vi "USB6343_Control_v1.6.vi"(8 "error in":errorcluster caption="错误输出") -> (0 "error out":errorcluster caption="错误输出")   [LabVIEW 2013]
uses:
  <vilib>/DAQmx/read.llb/DAQmx Read (Analog 1D DBL NChan 1Samp).vi
  <vilib>/DAQmx/read.llb/DAQmx Read (Digital 1D Bool NChan 1Samp 1Line).vi
  <vilib>/DAQmx/read.llb/DAQmx Read (Counter DBL 1Chan 1Samp).vi
  <vilib>/DAQmx/write.llb/DAQmx Write (Digital 1D Bool NChan 1Samp 1Line).vi
  <vilib>/DAQmx/write.llb/DAQmx Write (Analog 1D DBL NChan 1Samp).vi
  <vilib>/DAQmx/miscellaneous.llb/DAQmx Fill In Error Info.vi
  current_position.vi
  <vilib>/DAQmx/configure/timing.llb/DAQmx Timing (Implicit).vi
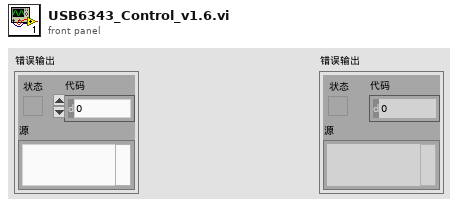
[diagram p1: front panel]
types:
  T1 = typedef "Semaphore RefNum" = refnum<k1>
  T2 = cluster{"monitor":refnum<user-event>, "motor status":refnum<user-event>, "motor":refnum<user-event>, "notifier out":refnum<notifier>, "queue out":refnum<queue>, "AI":T1, "DI":T1, "CX":T1, "CY":T1}
  T3 = cluster{"AI Task":refnum<k21>, "AO Task":refnum<k21>, "DO Task":refnum<k21>, "DI Task":refnum<k21>, "PWM x":refnum<k21>, "PWM y":refnum<k21>, "counter x":refnum<k21>, "counter y":refnum<k21>}
  T4 = cluster{"cmd":string, "channel":i32, "value":dbl, "on/off":bool, "return value":refnum<vi>}
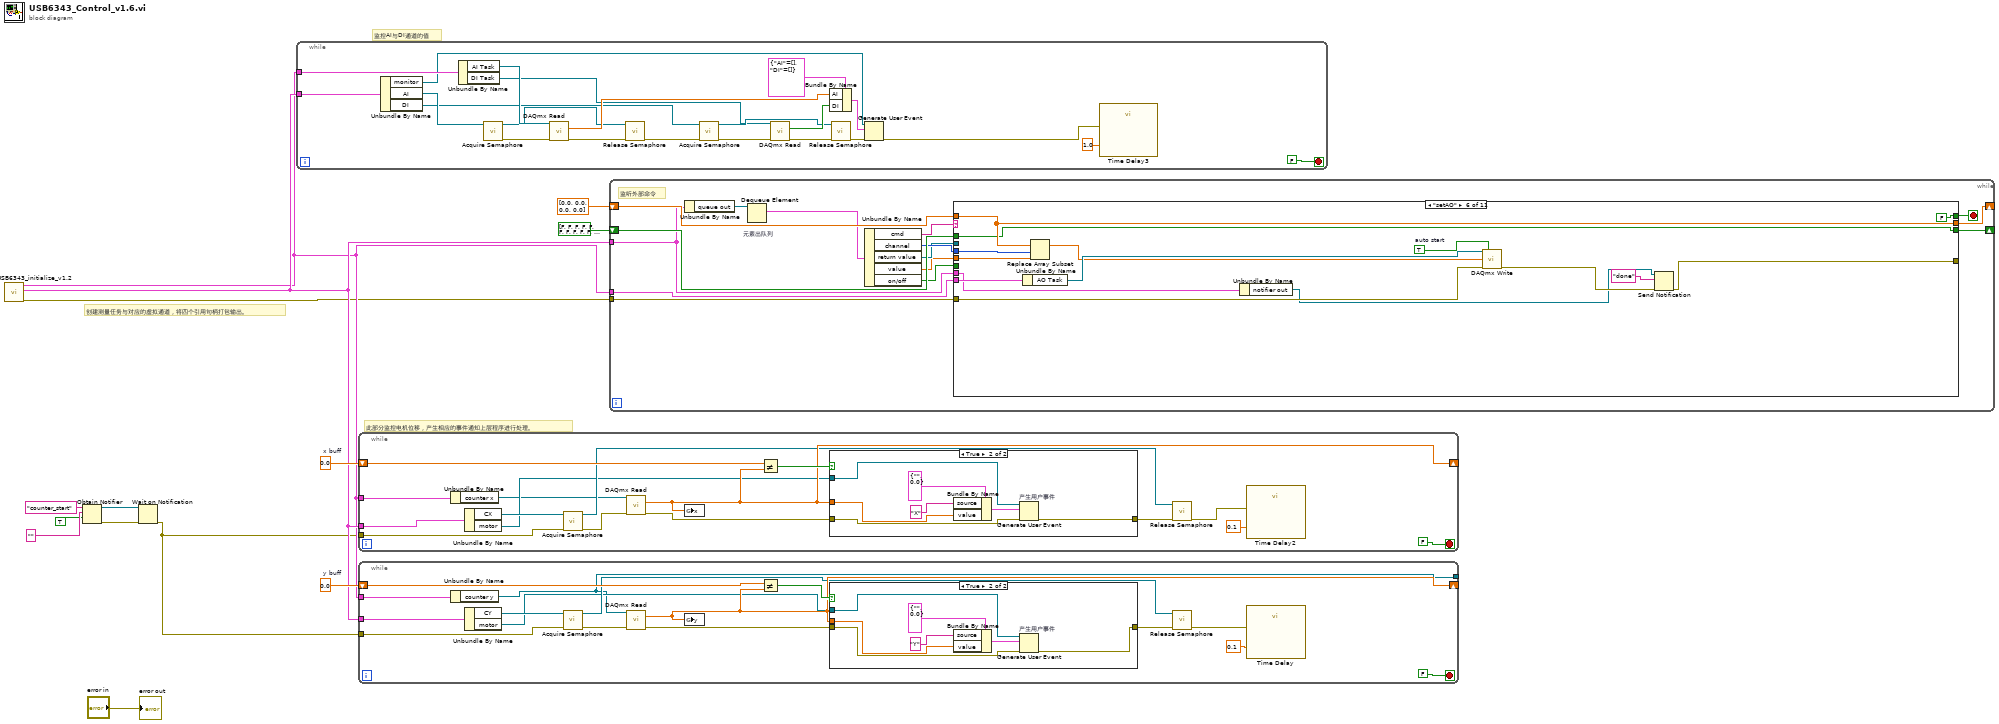
[diagram p0: block diagram]
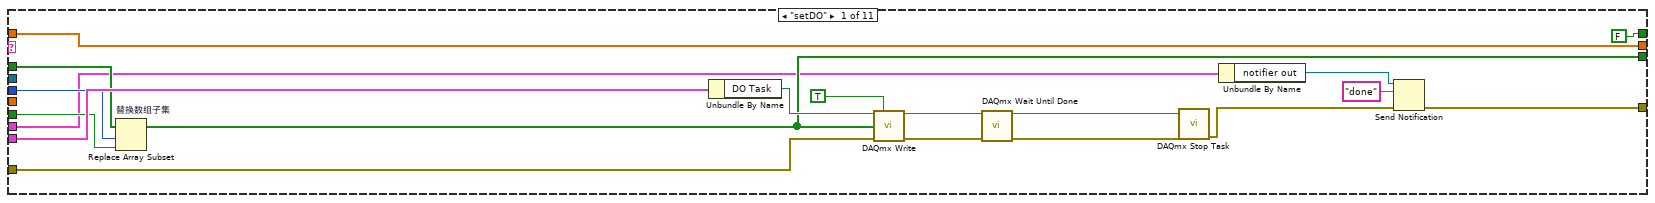
[diagram p4: hidden frame]
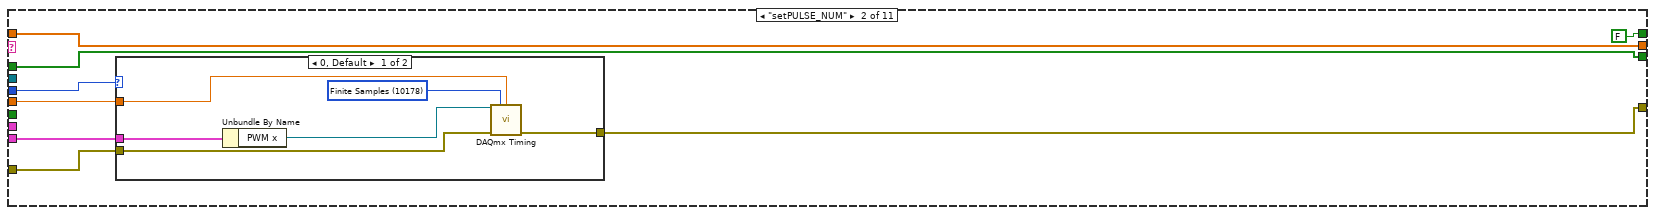
[diagram p5: hidden frame]
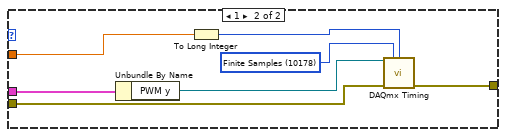
[diagram p6: hidden frame]
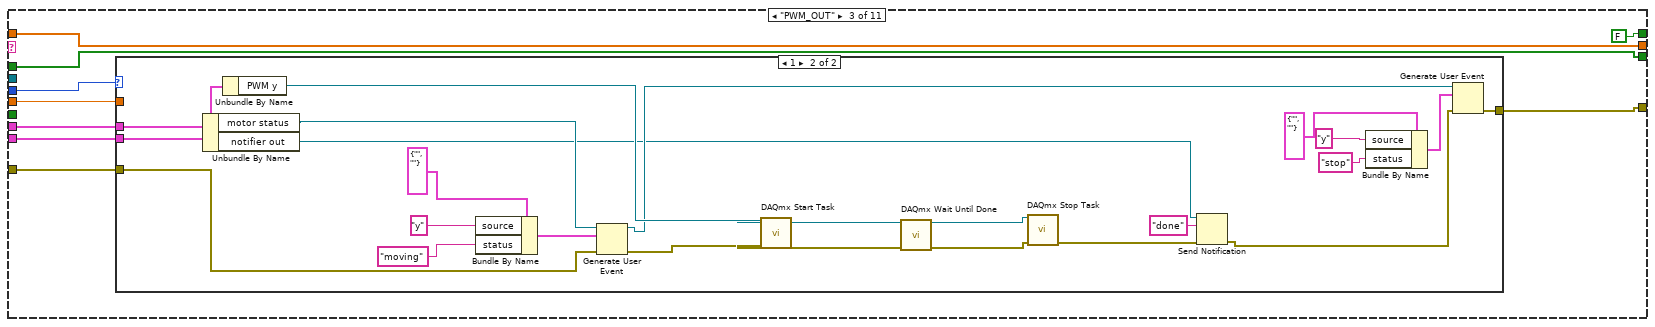
[diagram p7: hidden frame]
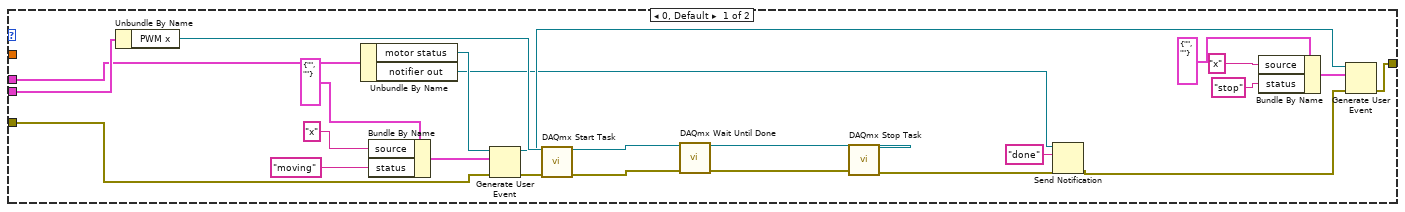
[diagram p8: hidden frame]
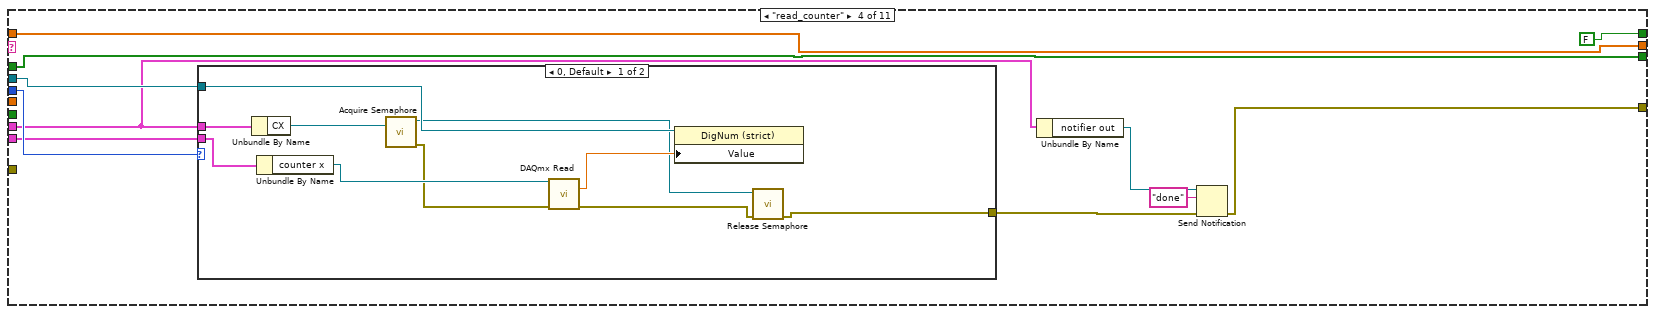
[diagram p9: hidden frame]
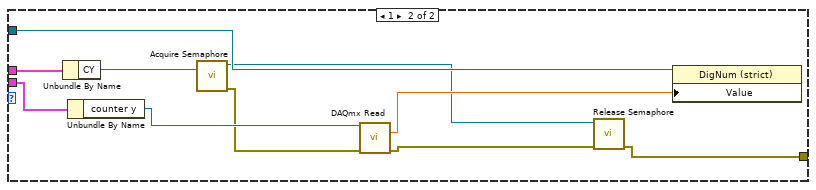
[diagram p10: hidden frame]
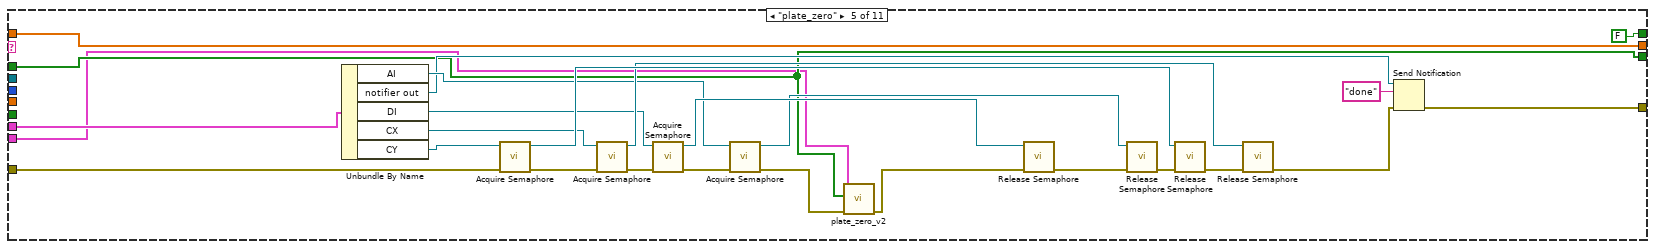
[diagram p11: hidden frame]
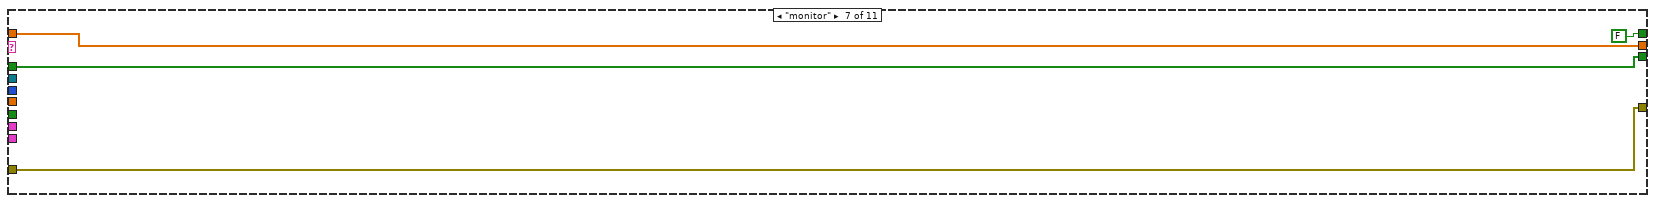
[diagram p12: hidden frame]
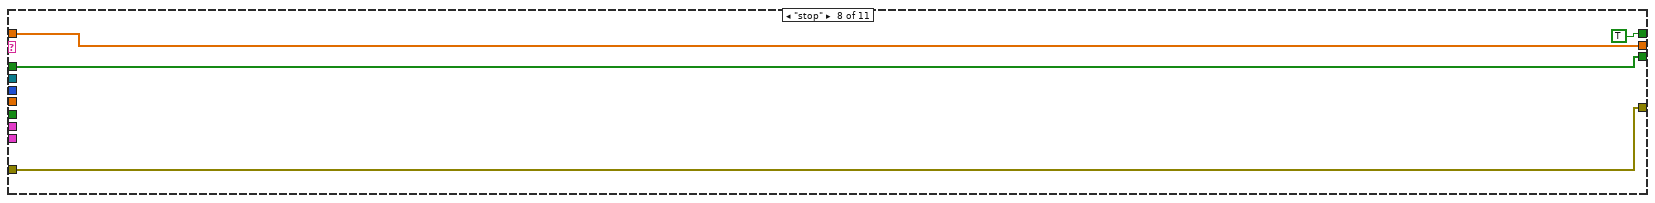
[diagram p13: hidden frame]
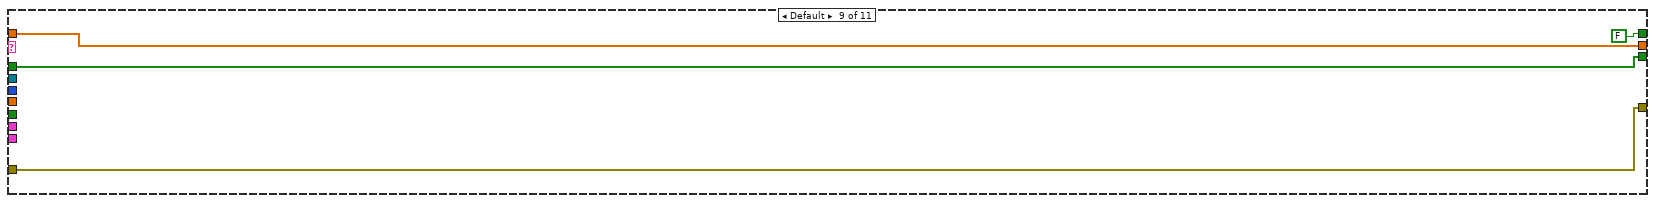
[diagram p14: hidden frame]
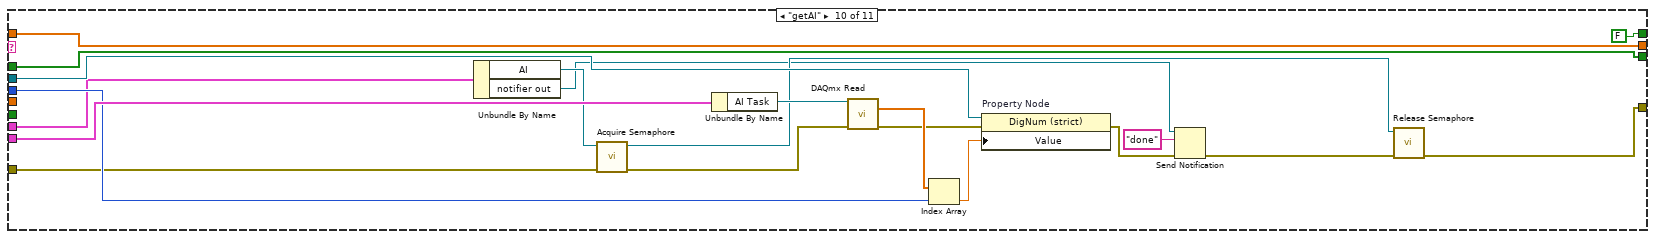
[diagram p15: hidden frame]
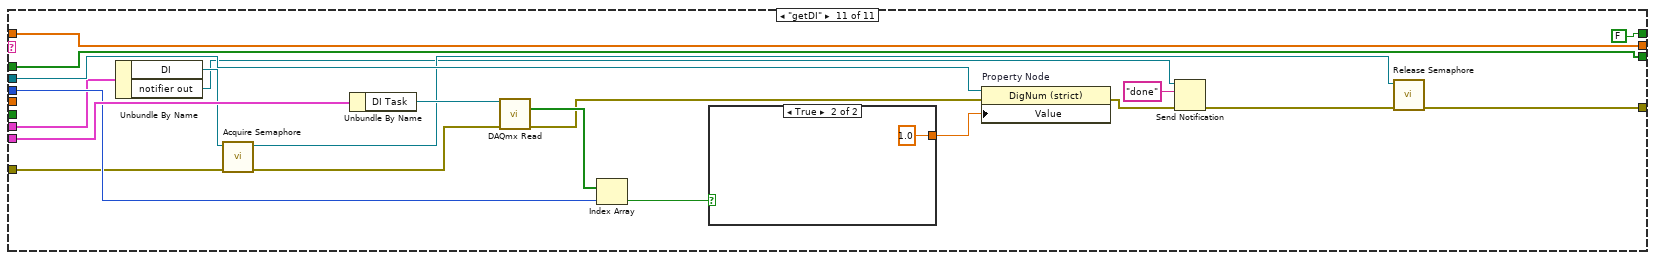
[diagram p16: hidden frame]
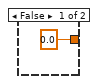
[diagram p17: hidden frame]
diagram:
  w11 = 0.0  # x buff
  w12 = 0.0  # y buff
  # "监控AI与DI通道的值"
  # "此部分监控电机位移，产生相应的事件通知上层程序进行处理。"
  # "创建测量任务与对应的虚拟通道，将四个引用句柄打包输出。"
  n1 = call "USB6343_initialize_v1.2.vi"() -> ("error out"=w7:errorcluster, "interface"=w10:T2, "tasks"=w9:T3)  [unwired: 9 in]
  n2 = Obtain Notifier(name (unnamed)="counter_start", notification data type="", create if not found? (T)=TRUE) -> (notifier out=w3:refnum<notifier>, error out=w4:errorcluster)  [unwired: 1 in, 1 out]
  n3 = Wait on Notification(notifier=w3, error in (no error)=w4) -> (error out=w2:errorcluster)  [unwired: 2 in, 3 out]
  n4 = while {
    tunnel: w9 -> [w34]
    tunnel: w10 -> [w19]
    stop <- FALSE stop-if-true
    n5 = Unbundle By Name(w19) -> ("monitor"=w18:refnum<user-event>, "AI"=w17:T1, "DI"=w16:T1)
    n6 = Unbundle By Name(w34) -> ("AI Task"=w35:refnum<k21>, "DI Task"=w15:refnum<k21>)
    n7 = call <vilib>:"Acquire Semaphore.vi"("semaphore"=w17) -> ("error out"=w20:errorcluster, "semaphore out"=w22:T1)  [unwired: 4 in, 1 out]
    n8 = call-poly <vilib>:"DAQmx Read.vi"("task/channels in"=w35, "error in"=w20) -> ("data"=w32:dbl[], "error out"=w27:errorcluster)  [unwired: 11 in, 1 out]
    n9 = call <vilib>:"Release Semaphore.vi"("error in (no error)"=w27, "semaphore"=w22) -> ("error out"=w26:errorcluster)  [unwired: 4 in, 1 out]
    n10 = call <vilib>:"Acquire Semaphore.vi"("error in (no error)"=w26, "semaphore"=w16) -> ("error out"=w25:errorcluster, "semaphore out"=w21:T1)  [unwired: 3 in, 1 out]
    n11 = call-poly <vilib>:"DAQmx Read.vi"("task/channels in"=w15, "error in"=w25) -> ("data"=w31:bool[], "error out"=w24:errorcluster)  [unwired: 11 in, 1 out]
    n12 = Bundle By Name(cluster=cluster{"AI":dbl[], "DI":bool[]} {"AI"=[], "DI"=[]} ("event data"), "AI"=w32, "DI"=w31) -> (w28:cluster{"AI":dbl[], "DI":bool[]})
    n13 = call <vilib>:"Release Semaphore.vi"("error in (no error)"=w24, "semaphore"=w21) -> ("error out"=w23:errorcluster)  [unwired: 4 in, 1 out]
    n14 = Generate User Event(user event=w18, event data cluster=w28, error in=w23) -> (error out=w30:errorcluster)  [unwired: 1 in, 1 out]
    n15 = call "Time Delay3"("error in (no error)"=w30, "Delay Time (s)"=1.0) -> ()  [unwired: 9 in, 1 out]
  }
  n16 = while {
    shift-right: [w48] -> _
    shift-left: w11 -> [w52]
    tunnel: w10 -> [w42]
    tunnel: w9 -> [w39]
    tunnel: w2 -> [w37]
    stop <- FALSE stop-if-true
    n17 = Unbundle By Name(w39) -> ("counter x"=w38:refnum<k21>)
    n18 = Unbundle By Name(w42) -> ("CX"=w41:T1, "motor"=w40:refnum<user-event>)
    n19 = call <vilib>:"Acquire Semaphore.vi"("error in (no error)"=w37, "semaphore"=w41) -> ("error out"=w47:errorcluster, "semaphore out"=w44:T1)  [unwired: 3 in, 1 out]
    n20 = call-poly <vilib>:"DAQmx Read.vi"("task/channels in"=w38, "error in"=w47) -> ("data"=w48:dbl, "error out"=w50:errorcluster)  [unwired: 11 in, 1 out]
    n21 = global write "current_position.vi" "x"(w48) -> ()
    n22 = Not Equal?(x=w52, y=w48) -> (x != y?=w51:bool)
    n23 = case shown="True" w51 {
      tunnel: w48 -> [_ w54]
      tunnel: w50 -> [w53 w57]
      tunnel: [w53 w56] -> w46
      tunnel: w40 -> [_ w55]
      frame False {
      }
      frame True {
        n24 = Bundle By Name(cluster=cluster{"source":string, "value":dbl} {"source"="", "value"=0.0} ("事件数据"), "source"="X", "value"=w54) -> (w58:cluster{"source":string, "value":dbl})
        n25 = Generate User Event "产生用户事件"(user event=w55, event data cluster=w58, error in=w57) -> (error out=w56:errorcluster)  [unwired: 1 in, 1 out]
      }
    }
    n26 = call <vilib>:"Release Semaphore.vi"("error in (no error)"=w46, "semaphore"=w44) -> ("error out"=w45:errorcluster)  [unwired: 4 in, 1 out]
    n27 = call "Time Delay2"("error in (no error)"=w45, "Delay Time (s)"=0.1) -> ()  [unwired: 9 in, 1 out]
  }
  n28 = while {
    tunnel: [w62] -> _
    shift-right: [w72] -> _
    shift-left: w12 -> [w76]
    tunnel: w10 -> [w66]
    tunnel: w9 -> [w63]
    tunnel: w2 -> [w61]
    stop <- FALSE stop-if-true
    n29 = Unbundle By Name(w63) -> ("counter y"=w62:refnum<k21>)
    n30 = Unbundle By Name(w66) -> ("CY"=w65:T1, "motor"=w64:refnum<user-event>)
    n31 = call <vilib>:"Acquire Semaphore.vi"("error in (no error)"=w61, "semaphore"=w65) -> ("error out"=w71:errorcluster, "semaphore out"=w68:T1)  [unwired: 3 in, 1 out]
    n32 = call-poly <vilib>:"DAQmx Read.vi"("task/channels in"=w62, "error in"=w71) -> ("data"=w72:dbl, "error out"=w74:errorcluster)  [unwired: 11 in, 1 out]
    n33 = global write "current_position.vi" "y"(w72) -> ()
    n34 = Not Equal?(x=w76, y=w72) -> (x != y?=w75:bool)
    n35 = case shown="True" w75 {
      tunnel: w72 -> [_ w78]
      tunnel: w74 -> [w77 w80]
      tunnel: [w77 w79] -> w70
      tunnel: w64 -> [_ w81]
      frame False {
      }
      frame True {
        n36 = Bundle By Name(cluster=cluster{"source":string, "value":dbl} {"source"="", "value"=0.0} ("事件数据"), "source"="Y", "value"=w78) -> (w82:cluster{"source":string, "value":dbl})
        n37 = Generate User Event "产生用户事件"(user event=w81, event data cluster=w82, error in=w80) -> (error out=w79:errorcluster)  [unwired: 1 in, 1 out]
      }
    }
    n38 = call <vilib>:"Release Semaphore.vi"("error in (no error)"=w70, "semaphore"=w68) -> ("error out"=w69:errorcluster)  [unwired: 4 in, 1 out]
    n39 = call "Time Delay"("error in (no error)"=w69, "Delay Time (s)"=0.1) -> ()  [unwired: 9 in, 1 out]
  }
  n40 = while {
    tunnel: w9 -> [w93]
    tunnel: w7 -> [w99]
    shift-right: [w97] -> _
    shift-left: bool[] [FALSE, FALSE, FALSE, FALSE, FALSE, FALSE, FALSE, FALSE, FALSE, FALSE, FALSE, FALSE, FALSE, FALSE, FALSE, FALSE] -> [w98]
    shift-right: [w94] -> _
    shift-left: dbl[] [0.0, 0.0, 0.0, 0.0] ("data") -> [w95]
    tunnel: w10 -> [w86]
    stop <- w96 stop-if-true
    # "监听外部命令"
    n41 = Unbundle By Name(w86) -> ("queue out"=w85:refnum<queue>)
    n42 = Dequeue Element "元素出队列"(queue=w85) -> (element=w92:T4)  [unwired: 2 in, 3 out]
    n43 = Unbundle By Name(w92) -> ("cmd"=w91:string, "channel"=w90:i32, "return value"=w89:refnum<vi>, "value"=w87:dbl, "on/off"=w88:bool)
    n44 = case shown="\"setAO\"" w91 {
      tunnel: w90 -> [w116 w120 w142 w207 _ w266 _ _ _ w296 w319]
      tunnel: w93 -> [w118 w123 w145 w206 w229 w268 _ _ _ w300 w321]
      tunnel: w99 -> [w110 w121 w143 _ w245 w260 w269 w273 w277 w289 w309]
      tunnel: w98 -> [w117 w124 w146 w197 w231 w264 w272 w276 w280 w294 w318]
      tunnel: w88 -> [w115 _ _ _ _ _ _ _ _ _ _]
      tunnel: [w108 w124 w146 w197 w231 w264 w272 w276 w280 w294 w318] -> w97
      tunnel: [FALSE FALSE FALSE FALSE FALSE FALSE FALSE TRUE FALSE FALSE FALSE] -> w96
      tunnel: w95 -> [w113 w125 w147 w198 w252 w265 w271 w274 w278 w293 w317]
      tunnel: [w113 w125 w147 w198 w252 w265 w271 w274 w278 w293 w317] -> w94
      tunnel: w89 -> [_ _ _ w205 _ _ _ _ _ w298 w320]
      tunnel: [w112 w119 w141 w200 w251 w257 w269 w273 w277 w285 w304] -> _
      tunnel: w87 -> [_ w122 w144 _ _ w259 _ _ _ _ _]
      tunnel: w86 -> [w104 _ w140 w203 w237 w256 _ _ _ w283 w303]
      frame "setDO" {
        n45 = Replace Array Subset "替换数组子集"(array=w117, new element=w115, index=w116) -> (w108:bool[])
        n46 = Unbundle By Name(w118) -> ("DO Task"=w109:refnum<k21>)
        n47 = call-poly <vilib>:"DAQmx Write.vi"("task/channels in"=w109, "auto start"=TRUE, "data"=w108, "error in"=w110) -> ("task out"=w105:refnum<k21>, "error out"=w106:errorcluster)  [unwired: 9 in, 1 out]
        n48 = call <vilib>:"DAQmx Wait Until Done.vi"("task/channels in"=w105, "error in"=w106) -> ("task out"=w100:refnum<k21>, "error out"=w102:errorcluster)  [unwired: 12 in]
        n49 = call <vilib>:"DAQmx Stop Task.vi"("task/channels in"=w100, "error in"=w102) -> ("error out"=w101:errorcluster)  [unwired: 12 in, 1 out]
        n50 = Unbundle By Name(w104) -> ("notifier out"=w103:refnum<notifier>)
        n51 = Send Notification(notification="done" ("通知"), notifier=w103, error in (no error)=w101) -> (error out=w112:errorcluster)  [unwired: 1 out]
      }
      frame "setPULSE_NUM" {
        n52 = case shown="0, Default" w120 {
          tunnel: w123 -> [w132 w139]
          tunnel: w122 -> [w129 w134]
          tunnel: w121 -> [w128 w136]
          tunnel: [w127 w135] -> w119
          frame 0, Default {
            w130 = 10178 items=["Finite Samples"=10178, "Continuous Samples"=10123, "Hardware Timed Single Point"=12522] ("sample mode")
            n53 = Unbundle By Name(w132) -> ("PWM x"=w131:refnum<k21>)
            n54 = call-poly <vilib>:"DAQmx Timing.vi"("task/channels in"=w131, "sample mode"=w130, "samples per channel"=w129, "error in"=w128) -> ("error out"=w127:errorcluster)  [unwired: 10 in, 1 out]
          }
          frame 1 {
            w137 = 10178 items=["Finite Samples"=10178, "Continuous Samples"=10123, "Hardware Timed Single Point"=12522] ("sample mode")
            n55 = Unbundle By Name(w139) -> ("PWM y"=w138:refnum<k21>)
            n56 = To Long Integer(number=w134) -> (32bit integer=w133:i32)
            n57 = call-poly <vilib>:"DAQmx Timing.vi"("task/channels in"=w138, "sample mode"=w137, "samples per channel"=w133, "error in"=w136) -> ("error out"=w135:errorcluster)  [unwired: 10 in, 1 out]
          }
        }
      }
      frame "PWM_OUT" {
        n58 = case shown="1" w142 {
          tunnel: w145 -> [w172 w196]
          tunnel: w144 -> [_ _]
          tunnel: w143 -> [w164 w188]
          tunnel: [w157 w182] -> w141
          tunnel: w140 -> [w155 w179]
          frame 0, Default {
            n59 = Unbundle By Name(w172) -> ("PWM x"=w171:refnum<k21>)
            n60 = Unbundle By Name(w155) -> ("motor status"=w154:refnum<user-event>, "notifier out"=w149:refnum<notifier>)
            n61 = Bundle By Name(cluster=cluster{"source":string, " status":string} {"source"="", " status"=""} ("event data"), "source"="x", "status"="moving") -> (w162:cluster{"source":string, " status":string})
            n62 = Generate User Event(user event=w154, event data cluster=w162, error in=w164) -> (user event out=w156:refnum<user-event>, error out=w163:errorcluster)  [unwired: 1 in]
            n63 = call <vilib>:"DAQmx Start Task.vi"("task/channels in"=w171, "error in"=w163) -> ("task out"=w169:refnum<k21>, "error out"=w170:errorcluster)  [unwired: 12 in]
            n64 = call <vilib>:"DAQmx Wait Until Done.vi"("task/channels in"=w169, "error in"=w170) -> ("task out"=w168:refnum<k21>, "error out"=w153:errorcluster)  [unwired: 12 in]
            n65 = call <vilib>:"DAQmx Stop Task.vi"("task/channels in"=w168, "error in"=w153) -> ("error out"=w152:errorcluster)  [unwired: 12 in, 1 out]
            n66 = Send Notification(notification="done", notifier=w149, error in (no error)=w152) -> (error out=w151:errorcluster)  [unwired: 1 out]
            n67 = Bundle By Name(cluster=cluster{"source":string, " status":string} {"source"="", " status"=""} ("event data"), "source"="x", "status"="stop") -> (w158:cluster{"source":string, " status":string})
            n68 = Generate User Event(user event=w156, event data cluster=w158, error in=w151) -> (error out=w157:errorcluster)  [unwired: 1 in, 1 out]
          }
          frame 1 {
            n69 = Unbundle By Name(w179) -> ("motor status"=w178:refnum<user-event>, "notifier out"=w173:refnum<notifier>)
            n70 = Unbundle By Name(w196) -> ("PWM y"=w195:refnum<k21>)
            n71 = Bundle By Name(cluster=cluster{"source":string, " status":string} {"source"="", " status"=""} ("event data"), "source"="y", "status"="moving") -> (w181:cluster{"source":string, " status":string})
            n72 = Generate User Event(user event=w178, event data cluster=w181, error in=w188) -> (user event out=w177:refnum<user-event>, error out=w187:errorcluster)  [unwired: 1 in]
            n73 = call <vilib>:"DAQmx Start Task.vi"("task/channels in"=w195, "error in"=w187) -> ("task out"=w193:refnum<k21>, "error out"=w194:errorcluster)  [unwired: 12 in]
            n74 = call <vilib>:"DAQmx Wait Until Done.vi"("task/channels in"=w193, "error in"=w194) -> ("task out"=w191:refnum<k21>, "error out"=w192:errorcluster)  [unwired: 12 in]
            n75 = call <vilib>:"DAQmx Stop Task.vi"("task/channels in"=w191, "error in"=w192) -> ("error out"=w176:errorcluster)  [unwired: 12 in, 1 out]
            n76 = Send Notification(notification="done", notifier=w173, error in (no error)=w176) -> (error out=w175:errorcluster)  [unwired: 1 out]
            n77 = Bundle By Name(cluster=cluster{"source":string, " status":string} {"source"="", " status"=""} ("event data"), "source"="y", "status"="stop") -> (w183:cluster{"source":string, " status":string})
            n78 = Generate User Event(user event=w177, event data cluster=w183, error in=w175) -> (error out=w182:errorcluster)  [unwired: 1 in, 1 out]
          }
        }
      }
      frame "read_counter" {
        n79 = case shown="0, Default" w207 {
          tunnel: w203 -> [w217 w227]
          tunnel: w206 -> [w215 w225]
          tunnel: w205 -> [w212 w222]
          tunnel: [w208 w218] -> w204
          frame 0, Default {
            n80 = Unbundle By Name(w217) -> ("CX"=w216:T1)
            n81 = Unbundle By Name(w215) -> ("counter x"=w214:refnum<k21>)
            n82 = call <vilib>:"Acquire Semaphore.vi"("semaphore"=w216) -> ("error out"=w213:errorcluster, "semaphore out"=w209:T1)  [unwired: 4 in, 1 out]
            n83 = call-poly <vilib>:"DAQmx Read.vi"("task/channels in"=w214, "error in"=w213) -> ("data"=w211:dbl, "error out"=w210:errorcluster)  [unwired: 11 in, 1 out]
            n84 = property class="DigNum (strict)"(reference=w212, "Value"=w211) -> ()  [unwired: 1 in, 2 out]
            n85 = call <vilib>:"Release Semaphore.vi"("error in (no error)"=w210, "semaphore"=w209) -> ("error out"=w208:errorcluster)  [unwired: 4 in, 1 out]
          }
          frame 1 {
            n86 = Unbundle By Name(w227) -> ("CY"=w226:T1)
            n87 = Unbundle By Name(w225) -> ("counter y"=w224:refnum<k21>)
            n88 = call <vilib>:"Acquire Semaphore.vi"("semaphore"=w226) -> ("error out"=w223:errorcluster, "semaphore out"=w219:T1)  [unwired: 4 in, 1 out]
            n89 = call-poly <vilib>:"DAQmx Read.vi"("task/channels in"=w224, "error in"=w223) -> ("data"=w221:dbl, "error out"=w220:errorcluster)  [unwired: 11 in, 1 out]
            n90 = call <vilib>:"Release Semaphore.vi"("error in (no error)"=w220, "semaphore"=w219) -> ("error out"=w218:errorcluster)  [unwired: 4 in, 1 out]
            n91 = property class="DigNum (strict)"(reference=w222, "Value"=w221) -> ()  [unwired: 1 in, 2 out]
          }
        }
        n92 = Unbundle By Name(w203) -> ("notifier out"=w202:refnum<notifier>)
        n93 = Send Notification(notification="done", notifier=w202, error in (no error)=w204) -> (error out=w200:errorcluster)  [unwired: 1 out]
      }
      frame "plate_zero" {
        n94 = Unbundle By Name(w237) -> ("AI"=w236:T1, "notifier out"=w232:refnum<notifier>, "DI"=w235:T1, "CX"=w234:T1, "CY"=w233:T1)
        n95 = call <vilib>:"Acquire Semaphore.vi"("error in (no error)"=w245, "semaphore"=w233) -> ("error out"=w247:errorcluster, "semaphore out"=w241:T1)  [unwired: 3 in, 1 out]
        n96 = call <vilib>:"Acquire Semaphore.vi"("error in (no error)"=w247, "semaphore"=w234) -> ("error out"=w246:errorcluster, "semaphore out"=w238:T1)  [unwired: 3 in, 1 out]
        n97 = call <vilib>:"Acquire Semaphore.vi"("error in (no error)"=w246, "semaphore"=w235) -> ("error out"=w249:errorcluster, "semaphore out"=w240:T1)  [unwired: 3 in, 1 out]
        n98 = call <vilib>:"Acquire Semaphore.vi"("error in (no error)"=w249, "semaphore"=w236) -> ("error out"=w230:errorcluster, "semaphore out"=w239:T1)  [unwired: 3 in, 1 out]
        n99 = call "plate_zero_v2.vi"("error in"=w230, "DO array"=w231, "tasks"=w229) -> ("error out"=w228:errorcluster)  [unwired: 8 in]
        n100 = call <vilib>:"Release Semaphore.vi"("error in (no error)"=w228, "semaphore"=w240) -> ("error out"=w248:errorcluster)  [unwired: 4 in, 1 out]
        n101 = call <vilib>:"Release Semaphore.vi"("error in (no error)"=w248, "semaphore"=w239) -> ("error out"=w244:errorcluster)  [unwired: 4 in, 1 out]
        n102 = call <vilib>:"Release Semaphore.vi"("error in (no error)"=w244, "semaphore"=w241) -> ("error out"=w243:errorcluster)  [unwired: 4 in, 1 out]
        n103 = call <vilib>:"Release Semaphore.vi"("error in (no error)"=w243, "semaphore"=w238) -> ("error out"=w242:errorcluster)  [unwired: 4 in, 1 out]
        n104 = Send Notification(notification="done", notifier=w232, error in (no error)=w242) -> (error out=w251:errorcluster)  [unwired: 1 out]
      }
      frame "setAO" {
        w262 = TRUE  # auto start
        n105 = Unbundle By Name(w268) -> ("AO Task"=w267:refnum<k21>)
        n106 = Replace Array Subset(array=w265, new element=w259, index=w266) -> (w263:dbl[])
        n107 = Unbundle By Name(w256) -> ("notifier out"=w255:refnum<notifier>)
        n108 = call-poly <vilib>:"DAQmx Write.vi"("task/channels in"=w267, "auto start"=w262, "data"=w263, "error in"=w260) -> ("error out"=w258:errorcluster)  [unwired: 9 in, 2 out]
        n109 = Send Notification(notification="done", notifier=w255, error in (no error)=w258) -> (error out=w257:errorcluster)  [unwired: 1 out]
      }
      frame "monitor" {
      }
      frame "stop" {
      }
      frame Default {
      }
      frame "getAI" {
        n110 = Unbundle By Name(w283) -> ("AI"=w282:T1, "notifier out"=w281:refnum<notifier>)
        n111 = call <vilib>:"Acquire Semaphore.vi"("error in (no error)"=w289, "semaphore"=w282) -> ("error out"=w288:errorcluster, "semaphore out"=w284:T1)  [unwired: 3 in, 1 out]
        n112 = Unbundle By Name(w300) -> ("AI Task"=w299:refnum<k21>)
        n113 = call-poly <vilib>:"DAQmx Read.vi"("task/channels in"=w299, "error in"=w288) -> ("data"=w297:dbl[], "error out"=w287:errorcluster)  [unwired: 11 in, 1 out]
        n114 = Index Array(array=w297, index=w296) -> (element=w295:dbl)
        n115 = property on="Property Node" class="DigNum (strict)"(reference=w298, error in=w287, "Value"=w295) -> (error out=w290:errorcluster)  [unwired: 1 out]
        n116 = Send Notification(notification="done" ("通知"), notifier=w281, error in (no error)=w290) -> (error out=w286:errorcluster)  [unwired: 1 out]
        n117 = call <vilib>:"Release Semaphore.vi"("error in (no error)"=w286, "semaphore"=w284) -> ("error out"=w285:errorcluster)  [unwired: 4 in, 1 out]
      }
      frame "getDI" {
        n118 = Unbundle By Name(w303) -> ("DI"=w302:T1, "notifier out"=w301:refnum<notifier>)
        n119 = call <vilib>:"Acquire Semaphore.vi"("error in (no error)"=w309, "semaphore"=w302) -> ("error out"=w308:errorcluster, "semaphore out"=w305:T1)  [unwired: 3 in, 1 out]
        n120 = Unbundle By Name(w321) -> ("DI Task"=w313:refnum<k21>)
        n121 = call-poly <vilib>:"DAQmx Read.vi"("task/channels in"=w313, "error in"=w308) -> ("data"=w312:bool[], "error out"=w307:errorcluster)  [unwired: 11 in, 1 out]
        n122 = Index Array "Index Array"(array=w312, index=w319) -> (element=w311:bool)
        n123 = case shown="True" w311 {
          tunnel: [0.0 1.0] -> w310
          frame False {
          }
          frame True {
          }
        }
        n124 = property on="Property Node" class="DigNum (strict)"(reference=w320, error in=w307, "Value"=w310) -> (error out=w314:errorcluster)  [unwired: 1 out]
        n125 = Send Notification(notification="done" ("通知"), notifier=w301, error in (no error)=w314) -> (error out=w306:errorcluster)  [unwired: 1 out]
        n126 = call <vilib>:"Release Semaphore.vi"("error in (no error)"=w306, "semaphore"=w305) -> ("error out"=w304:errorcluster)  [unwired: 4 in, 1 out]
      }
    }
  }
  "error out" <- "error in"
